vi "Status Channel GUID.vi"() -> (3 "Status GUID":string="5f2c7c82-531a-4580-8cae-6bebe0aabebf")   [LabVIEW 2019, in "DSF Shared.lvlib"]
uses:
  DSF Shared.lvlib
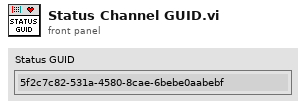
[diagram p1: front panel]
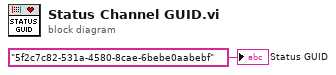
[diagram p0: block diagram]
diagram:
  "Status GUID" <- "5f2c7c82-531a-4580-8cae-6bebe0aabebf" ("Data Sharing Framework")
